vi "Print Front Panel.vi"(8 "error in (no error)":errorcluster, 10 "Front panel image path":path, 11 "VI in":refnum<vi>) -> (0 "error out":errorcluster)   [LabVIEW 2018]
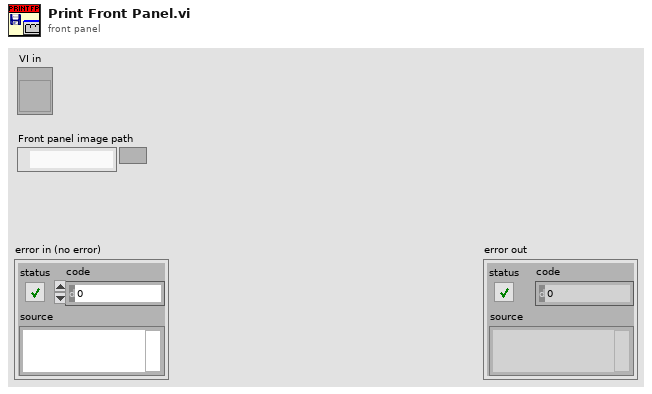
[diagram p1: front panel]
types:
  T1 = typedef "imagedata.ctl" = cluster{"image type":i32, "image depth":i32, "image":u8[], "mask":u8[], "colors":u32[], "Rectangle":cluster{"left":i16, "top":i16, "right":i16, "bottom":i16}}
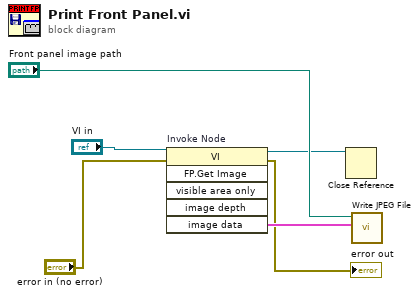
[diagram p0: block diagram]
diagram:
  n1 = invoke on="Invoke Node" class="VI" method="FP.Get Image"(reference="VI in", error in="error in (no error)") -> (reference out=w4:refnum<vi>, error out=→"error out":errorcluster, "image data"=w5:T1)  [unwired: 4 in, 3 out]
  n2 = Close Reference(reference=w4) -> ()  [unwired: 1 in, 1 out]
  n3 = call <vilib>:"Write JPEG File.vi"("image data"=w5, "path to JPEG file"="Front panel image path") -> ()  [unwired: 8 in, 2 out]
